vi "Test File Info FLAC.vi"(8 "error in (no error)":errorcluster) -> (0 "error out":errorcluster, 3 "Pass?":bool)   [LabVIEW 2020]
uses:
  G-Audio/Controls/Audio File Codec.ctl
  G-Audio/G-Audio.lvlib
  G-Audio/Controls/Audio File Info.ctl
  4dacca59-2375-4c52-b8d0-ae6ba5441d47.vi
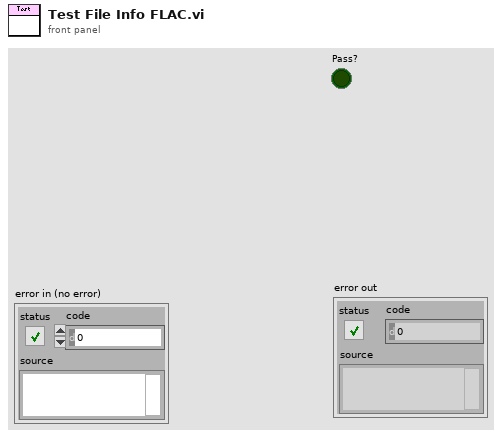
[diagram p1: front panel]
types:
  T1 = typedef "G-Audio.lvlib/Audio File Info.ctl" = cluster{"Sample Rate (Hz)":u32, "Channels":u32, "Bit Depth":u32}
  T2 = typedef "G-Audio.lvlib/Audio File Codec.ctl" = enum16{"flac", "mp3", "vorbis", "wav", "unsupported"}
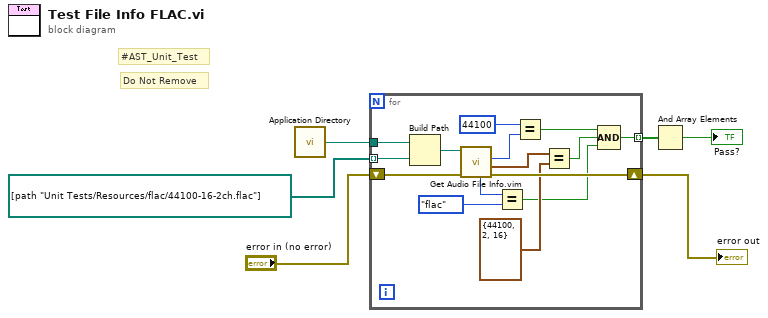
[diagram p0: block diagram]
diagram:
  # "Do Not Remove"
  # "#AST_Unit_Test"
  n1 = call <vilib>:"Application Directory.vi"() -> ("Application Directory"=w6:path)
  n2 = for {
    tunnel: w6 -> [w21]
    shift-right: [w19] -> w5
    shift-left: "error in (no error)" -> [w18]
    tunnel: path[] [path "Unit Tests/Resources/flac/44100-16-2ch.flac"] -> [w17] mode=indexing
    tunnel: [w7] -> w2 mode=indexing
    n3 = Build Path(base path=w21, name or relative path=w17) -> (appended path=w20:path)
    n4 = call "Get Audio File Info.vim"("error in (no error)"=w18, "Path In"=w20) -> ("error out"=w19:errorcluster, "Audio File Info"=w12:T1, "PCM Frame Length"=w14:u64, "Codec"=w16:T2)  [unwired: 5 in, 1 out]
    n5 = Equal?(x=w16, y=Audio_File_Codec."flac" ("x")) -> (x = y?=w10:bool)
    n6 = Equal?(x=u64 44100, y=w14) -> (x = y?=w8:bool)
    n7 = Equal?(x=w12, y=T1 {"Sample Rate (Hz)"=44100, "Channels"=2, "Bit Depth"=16} ("Audio File Info")) -> (x = y?=w9:bool)
    n8 = Compound Arithmetic op=AND(w8, w9, w10) -> (w7:bool)
  }
  "error out" <- w5
  n9 = And Array Elements(Boolean array=w2) -> (logical AND=→"Pass?":bool)
